vi "Table Value To 2D DBL.vi"(11 "Table Ref In":refnum<vi>) -> (1 "I64 Out":dbl[][](array[numeric]), 3 "Table Ref Out":refnum<vi>)   [LabVIEW 2024]
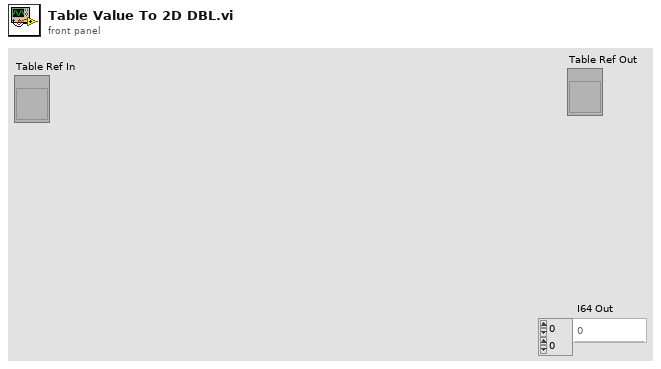
[diagram p1: front panel]
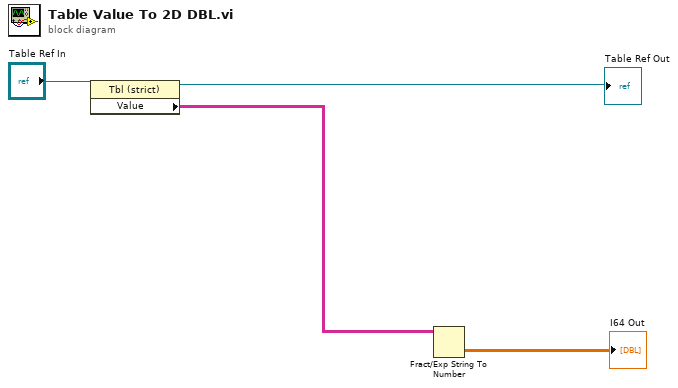
[diagram p0: block diagram]
diagram:
  n1 = property class="Tbl (strict)"(reference="Table Ref In") -> (reference out=→"Table Ref Out":refnum<vi>, "Value"=w2:string[][])  [unwired: 1 in, 1 out]
  n2 = Fract/Exp String To Number(string=w2) -> (number=→"I64 Out":dbl[][])  [unwired: 3 in, 1 out]
